vi "Write k_switch.vi"(8 "error in (no error)":errorcluster, 10 "k_switch":dbl, 11 "Ball in":refnum<class "Ball.lvclass">) -> (0 "error out":errorcluster, 3 "Ball out":refnum<class "Ball.lvclass">)   [LabVIEW 2023, in "Ball.lvclass"]
uses:
  Ball.lvclass
  Ball.lvclass/Ball.ctl
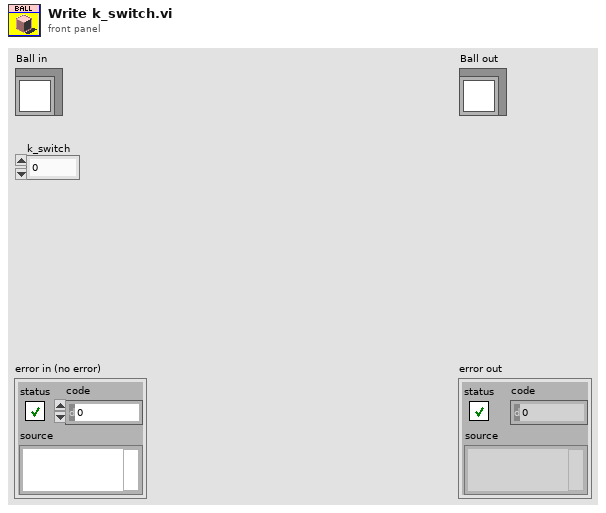
[diagram p1: front panel]
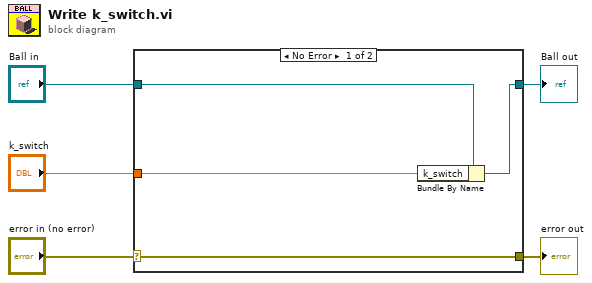
[diagram p0: block diagram]
diagram:
  n1 = case shown="No Error" "error in (no error)" {
    selector: "error in (no error)" -> [w9 w10]
    tunnel: [w9 w10] -> w4
    tunnel: [w7 w11] -> w2
    tunnel: "Ball in" -> [w8 w11]
    tunnel: "k_switch" -> [w6 _]
    frame No Error {
      n2 = Bundle By Name(cluster=w8, "k_switch"=w6) -> (w7:refnum<class "Ball.lvclass">)
    }
    frame Error {
    }
  }
  "error out" <- w4
  "Ball out" <- w2
